vi "Chroma ATE 6310 Mode Value Setup.vi"() -> ()   [LabVIEW 2015]
doc: "The getting started function shows how sub-VIs in CHROMA 6310 can be used.The general functions and modes can be used here.\n\nThis VI contains all modes and general configuration.In order to decrease the input items, the similar or same inputs from different modes are used in the same control panel.\nEx.: voltage level for CV mode, current level for CC mode and resistance level for CR mode can be controlled in the same panel \"Constant Level\"."
uses:
  <instrlib>/Chroma ATE 6310/Chroma ATE 6310.lvlib
panel:
  in  "Voltage Range(V) (16.0)":sgl=16.0 min=0 format="%.2f"
  in  "Von (1.0 V)":sgl=1.0 min=0 format="%.2f"
  out "VISA resource name out":refnum<visa-resource-name>
  out "error out":errorcluster
  in  "error in (no error)":errorcluster
  in  "VISA resource name":refnum<visa-resource-name>
  in  "Current Limit (0.0A)":sgl min=0 format="%.2f"
  in  "T2 (0.0)":sgl format="%.2f"
  in  "T1 (0.0)":sgl format="%.2f"
  in  "Fall (3.2)":sgl=3.2 min=0 step=0.32 format="%.2f"
  in  "Rise (3.2)":sgl=3.2 min=0 step=0.32 format="%.2f"
  in  "High/Low (1: High)":u32(slide)=1 scale=0.0..1.0
  in  "Static/Dynamic (0:Static)":u8(slide) scale=0.0..1.0
  in  "Mode (0:CC)":i8(slide) min=0 scale=0.0..2.0
  in  "Short (F:Off)":bool
  in  "Load (T: On)":bool=TRUE
  in  "Channel 1-8 (0:Ch1)":u8(ring) items=["Channel 1", "Channel 2", "Channel 3", "Channel 4", "Channel 5", "Channel 6", "Channel 7", "Channel 8 "]
  in  "Response Speed (1: Fast)":u8(slide) scale=0.0..1.0
  in  "Level 2 (0.0)":sgl min=0 format="%.4f"
  in  "Level 1 (5.0)":sgl=5.0 min=0 format="%.4f"
  # "© 2005 National Instruments.  ALL RIGHTS RESERVED."
  # "For CC Mode Only"
  # "On\nOff"
  # "On\nOff"
  # "For CV Mode Only"
  # "Constant Value"
  # "Slew Rate\n(mA/uS)"
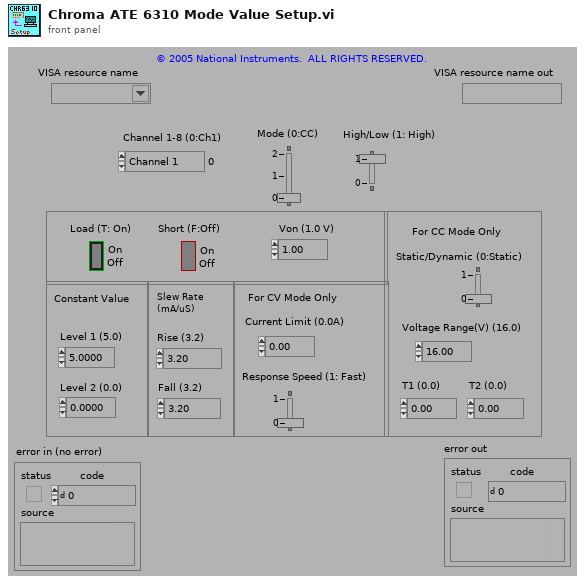
[diagram p1: front panel]
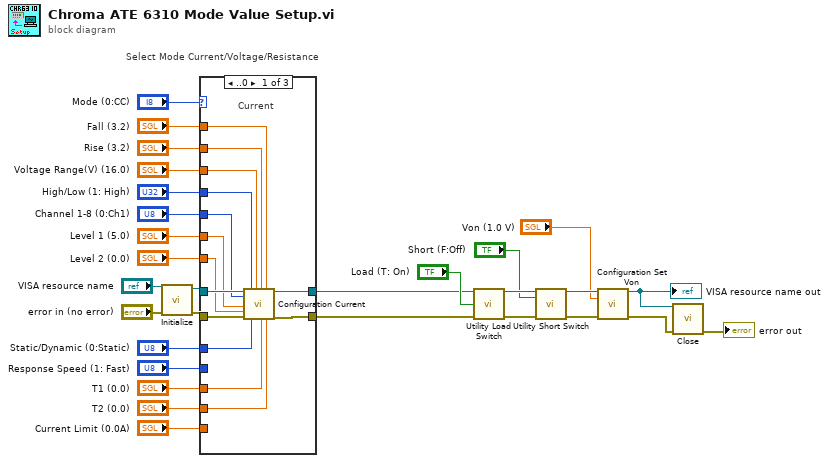
[diagram p0: block diagram]
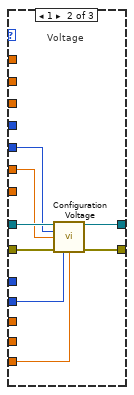
[diagram p2: hidden frame]
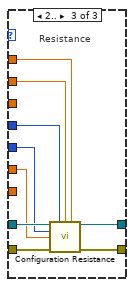
[diagram p3: hidden frame]
diagram:
  # "Select Mode Current/Voltage/Resistance"
  n1 = call <instrlib>:"Initialize.vi"("error in (no error)"="error in (no error)", "VISA resource name"="VISA resource name") -> ("error out"=w6:errorcluster, "VISA resource name out"=w4:refnum<visa-resource-name>)  [unwired: 8 in]
  n2 = case shown="..0" "Mode (0:CC)" {
    tunnel: [w43 w50 w60] -> w24
    tunnel: [w42 w51 w59] -> w25
    tunnel: w4 -> [w41 w48 w58]
    tunnel: w6 -> [w40 w49 w57]
    tunnel: "Channel 1-8 (0:Ch1)" -> [w39 w47 w56]
    tunnel: "Level 1 (5.0)" -> [w38 w46 w55]
    tunnel: "Level 2 (0.0)" -> [w37 _ _]
    tunnel: "High/Low (1: High)" -> [w36 _ w54]
    tunnel: "Rise (3.2)" -> [w35 _ w53]
    tunnel: "Fall (3.2)" -> [w34 _ w52]
    tunnel: "Static/Dynamic (0:Static)" -> [w33 _ _]
    tunnel: "T1 (0.0)" -> [w32 _ _]
    tunnel: "T2 (0.0)" -> [w31 _ _]
    tunnel: "Response Speed (1: Fast)" -> [_ w45 _]
    tunnel: "Current Limit (0.0A)" -> [_ w44 _]
    tunnel: "Voltage Range(V) (16.0)" -> [w30 _ _]
    frame ..0 {
      # "Current"
      n3 = call <instrlib>:"Configuration Current.vi"("VISA resource name"=w41, "Channel 1-8 (0:Ch1)"=w39, "Level 1 (5.0)"=w38, "Level 2 (0.0)"=w37, "error in (no error)"=w40, "High/Low (1:High)"=w36, "Static/Dynamic (0:Static)"=w33, "Voltage Range(V) (16.0)"=w30, "Rise (3.2)"=w35, "T1 (0.0)"=w32, "Fall (3.2)"=w34, "T2 (0.0)"=w31) -> ("VISA resource name out"=w42:refnum<visa-resource-name>, "error out"=w43:errorcluster)  [unwired: 6 in]
    }
    frame 1 {
      # "Voltage"
      n4 = call <instrlib>:"Configuration Voltage.vi"("VISA resource name"=w48, "Channel 1-8 (0:Ch1)"=w47, "Voltage Level (40.0V)"=w46, "error in (no error)"=w49, "Response Speed (0:Slow)"=w45, "Current Limit (2.0A)"=w44) -> ("VISA resource name out"=w51:refnum<visa-resource-name>, "error out"=w50:errorcluster)  [unwired: 8 in]
    }
    frame 2.. {
      # "Resistance"
      n5 = call <instrlib>:"Configuration Resistance.vi"("VISA resource name"=w58, "High/Low (1:High)"=w54, "Rise (3.2)"=w53, "Fall (3.2)"=w52, "Channel 1-8 (0:Ch1)"=w56, "Resistance Level (7.5 Ohm)"=w55, "error in (no error)"=w57) -> ("VISA resource name out"=w59:refnum<visa-resource-name>, "error out"=w60:errorcluster)  [unwired: 7 in]
    }
  }
  n6 = call <instrlib>:"Utility Load Switch.vi"("VISA resource name"=w25, "Load (T: On)"="Load (T: On)", "error in (no error)"=w24) -> ("VISA resource name out"=w27:refnum<visa-resource-name>, "error out"=w26:errorcluster)  [unwired: 11 in]
  n7 = call <instrlib>:"Utility Short Switch.vi"("VISA resource name"=w27, "Short (F:Off)"="Short (F:Off)", "error in (no error)"=w26) -> ("VISA resource name out"=w12:refnum<visa-resource-name>, "error out"=w11:errorcluster)  [unwired: 11 in]
  n8 = call <instrlib>:"Configuration Set Von.vi"("VISA resource name"=w12, "Von (1.0 V)"="Von (1.0 V)", "error in (no error)"=w11) -> ("VISA resource name out"=w1:refnum<visa-resource-name>, "error out"=w3:errorcluster)  [unwired: 11 in]
  "VISA resource name out" <- w1
  n9 = call <instrlib>:"Close.vi"("VISA resource name"=w1, "error in (no error)"=w3) -> ("error out"=→"error out":errorcluster)  [unwired: 13 in]
